vi "General Aperiodic Triangle.vi"(5 "X":dbl[](array[numeric]), 6 "asymmetry":dbl=0.5 min=0.0 max=1.0, 7 "width":dbl=10.0, 8 "delta t":dbl=0.1, 9 "delay":dbl, 10 "amplitude":dbl=1.0, 11 "samples":i32=128) -> (0 "error":i32, 3 "Aperiod Triangle":dbl[](array[numeric]))   [LabVIEW 2014, in "NI_AALBase.lvlib"]
uses:
  NI_AALBase.lvlib
  lvanlys.dll
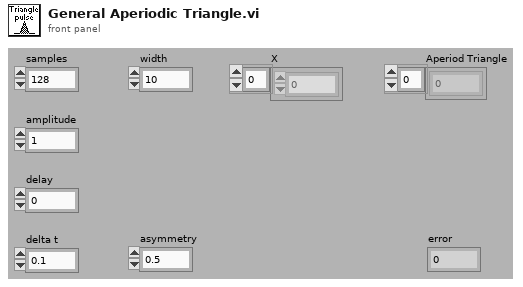
[diagram p1: front panel]
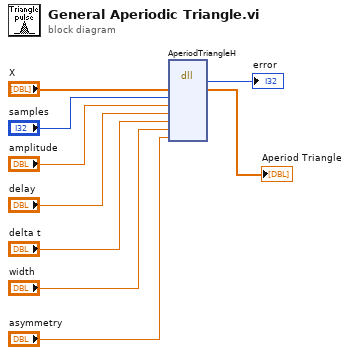
[diagram p0: block diagram]
diagram:
  n1 = dll-call lib="C:/Program Files (x86)/National Instruments/LabVIEW 2014/resource/lvanlys.*" fn="AperiodTriangleH"("x"="X", "samples"="samples", "amplitude"="amplitude", "delay"="delay", "delta"="delta t", "width"="width", "asymmetry"="asymmetry") -> ("error"=→"error":i32, "x"=→"Aperiod Triangle":dbl[])  [unwired: 9 in, 2 out]
